vi "Readable Demo.vi"() -> ()   [LabVIEW 2009]
uses:
  Dummy/Dummy.lvclass
panel:
  in  "Time per point":dbl[unit]=0.1
  out "TX graph":T1(graph)
  in  "stop":bool
  in  "Display last":dbl[unit]=10.0
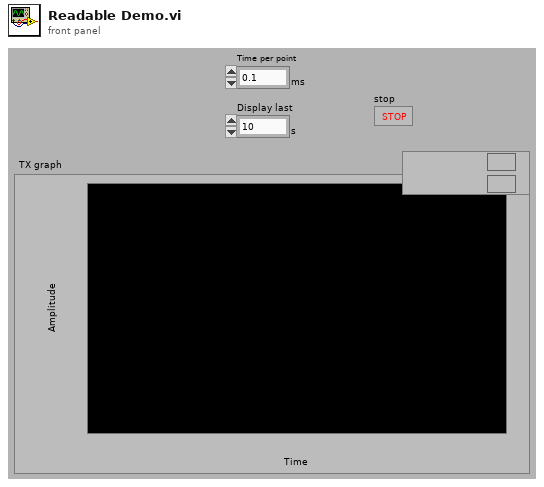
[diagram p1: front panel]
types:
  T1 = cluster{"Data Points":cluster{"t":timestamp, "x":dbl}[]}[]
  T2 = typedef "Readable.lvclass/TX Graph.ctl" = cluster{"Data Points":cluster{"t":timestamp, "x":dbl}[]}[]
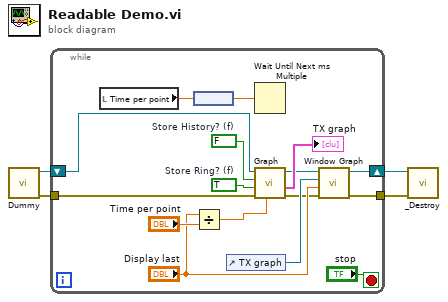
[diagram p0: block diagram]
diagram:
  n1 = call "Dummy.vi"() -> ("error out"=w4:errorcluster, "Dummy out"=w3:refnum<class "Dummy.lvclass">)  [unwired: 10 in]
  n2 = while {
    tunnel: w4 -> [w7]
    shift-right: [w10] -> w2
    shift-left: w3 -> [w12]
    tunnel: [w8] -> w1
    stop <- "stop" stop-if-true
    w6 = FALSE  # Store History? (f)
    w20 = TRUE  # Store Ring? (f)
    n3 = local read "Time per point"() -> (w5:dbl[unit])
    n4 = node(w5) -> (w17:dbl)
    n5 = Divide(x="Display last", y="Time per point") -> (x/y=w15:dbl)
    n6 = control-ref of="TX graph"() -> (w13:refnum<vi>)
    n7 = Wait Until Next ms Multiple(millisecond multiple=w17) -> ()  [unwired: 1 out]
    n8 = call-dynamic "Graph.vi"("Ring size (points) (1024)"=w15, "error in (no error)"=w7, "Store Ring? (f)"=w20, "Store History? (f)"=w6, "Readable in"=w12) -> ("error out"=w9:errorcluster, "Ring Buffers"=→"TX graph":T2, "Readable out"=w11:refnum<class "Dummy.lvclass">)  [unwired: 2 in, 2 out]
    n9 = call-dynamic "Window Graph.vi"("error in (no error)"=w9, "Window"="Display last", "Graph ref"=w13, "Readable in"=w11) -> ("error out"=w8:errorcluster, "Readable out"=w10:refnum<class "Dummy.lvclass">)  [unwired: 6 in]
  }
  n10 = call-dynamic "_Destroy.vi"("error in (no error)"=w1, "Instrument in"=w2) -> ()  [unwired: 9 in, 1 out]
